vi "UHR-Fleezers Control (host) - 12.5.vi"() -> ()   [LabVIEW 2012] (continued)
                  n249 = And(x=w462, y=w459) -> (x .and. y?=w461:bool)
                  n250 = case "Only if were fishing and now formed tether" shown="False" w461 {
                    tunnel: w460 -> [w464 w479]
                    tunnel: [w463 w478] -> w458
                    tunnel: w457 -> [_ w474]
                    frame False {
                      n251 = local read "Fish for Tether"() -> (w463:bool)
                      n252 = case shown="False" w463 {
                        tunnel: w464 -> [w465 _]
                        frame False {
                          n253 = property on="BD 1 Frequency 1 (MHz)" class="DigNum (strict)"("Val(Sgnl)"=w465) -> ()  [unwired: 2 in, 2 out]
                        }
                        frame True {
                        }
                      }
                    }
                    frame True {
                      w478 = FALSE ("Fish for Tether")
                      n254 = call <vilib>:"Beep.vi"() -> ()  [unwired: 3 in, 9 out]
                      n255 = Number To Decimal String(number=w474, width (-)=i16 1) -> (decimal integer string=w472:string)
                      n256 = Concatenate Strings("Formed tether in ", w472, " attempt(s)." ("string")) -> (w469:string)
                      n257 = local read "Messages"() -> (w476:string)
                      n258 = local write "Fish for Tether"(w478) -> ()
                      n259 = call "Update messages.vi"("Message to add"=w469, "Old message string"=w476) -> ("New message string"=w475:string)
                      n260 = local write "Messages"(w475) -> ()
                      n261 = Get Date/Time In Seconds() -> (seconds since 1Jan1904=→"Time tether formed":timestamp)
                      n262 = local read "Flow ON during cal?"() -> (w466:bool)
                      n263 = property on="Sample Channel\nFlow" class="Bool (strict)"("Val(Sgnl)"=w466) -> (error out=w467:errorcluster)  [unwired: 2 in, 1 out]
                      n264 = case shown="\"2\", \"3\", \"4\", \"5\", \"6\"" "Then..." {
                        selector: "Then..." -> [_ w482]
                        tunnel: w479 -> [w481 _]
                        tunnel: w467 -> [_ _]
                        frame "1", Default {
                          n265 = property on="BD 1 Frequency 1 (MHz)" class="DigNum (strict)"("Val(Sgnl)"=w481) -> ()  [unwired: 2 in, 2 out]
                        }
                        frame "2", "3", "4", "5", "6" {
                          n266 = flat-sequence {
                            tunnel: w482 -> [w484]
                            frame #0 {
                              n267 = property on="Trap Delta (MHz)" class="DigNum (strict)"("Val(Sgnl)"="Move to Delta 1 (MHz)") -> ()  [unwired: 2 in, 2 out]
                            }
                            frame #1 {
                              n268 = case shown="\"5\", \"6\"" w484 {
                                selector: w484 -> [w487 w497 _]
                                frame "3", "4" {
                                n269 = flat-sequence {
                                tunnel: w487 -> [w488]
                                tunnel: [w488] -> w485
                                tunnel: [w490] -> w486
                                tunnel: w485 -> [w490]
                                tunnel: w486 -> [w494]
                                frame #0 {
                                n270 = property on="Green Laser ON" class="Bool (strict)"("Val(Sgnl)"=TRUE ("Value (Signaling)")) -> ()  [unwired: 2 in, 2 out]
                                }
                                frame #1 {
                                n271 = Multiply(x="Wait Before Save (s)", y=u32 1000 ("x")) -> (x*y=w492:u32)
                                n272 = Wait (ms)(milliseconds to wait=w492) -> ()  [unwired: 1 out]
                                }
                                frame #2 {
                                n273 = property on="Start Saving" class="Bool (strict)"("Value"=TRUE ("Start Saving")) -> ()  [unwired: 2 in, 2 out]
                                n274 = case shown="\"4\"" w494 {
                                frame Default {
                                }
                                frame "4" {
                                n275 = property on="Fl. Triggered..." class="Bool (strict)"("Val(Sgnl)"=TRUE ("Value (Signaling)")) -> ()  [unwired: 2 in, 2 out]
                                }
                                }
                                }
                                }
                                }
                                frame "5", "6" {
                                n276 = stacked-sequence {
                                tunnel: w497 -> [_ _ _ _ _ _ w509]
                                frame #0 {
                                n277 = Replace Array Subset(array=u32[] [0] ("Index Values"), new element="Raster Set Upon Tether", index=0) -> (w498:u32[])
                                n278 = property on="Saved AOD Raster Scan Parameter Sets" class="Arr (strict)"("Index Values"=w498) -> ()  [unwired: 2 in, 2 out]
                                }
                                frame #1 {
                                n279 = Wait (ms)(milliseconds to wait=u32 500) -> ()  [unwired: 1 out]
                                }
                                frame #2 {
                                n280 = property on="Load parameters" class="Bool (strict)"("Val(Sgnl)"=TRUE ("Value (Signaling)")) -> ()  [unwired: 2 in, 2 out]
                                n281 = case shown="True" "Green ON During Raster" {
                                frame False {
                                }
                                frame True {
                                n282 = property on="Green Laser ON" class="Bool (strict)"("Val(Sgnl)"=TRUE ("Value (Signaling)")) -> ()  [unwired: 2 in, 2 out]
                                }
                                }
                                }
                                frame #3 {
                                n283 = Wait (ms)(milliseconds to wait=u32 500) -> ()  [unwired: 1 out]
                                }
                                frame #4 {
                                n284 = property on="Trap Raster Scan" class="Bool (strict)"("Val(Sgnl)"=TRUE ("Value (Signaling)")) -> ()  [unwired: 2 in, 2 out]
                                }
                                frame #5 {
                                n285 = Wait (ms)(milliseconds to wait=u32 2000) -> ()  [unwired: 1 out]
                                }
                                frame #6 {
                                n286 = flat-sequence {
                                tunnel: w509 -> [w516]
                                frame #0 {
                                n287 = while {
                                stop <- w512 stop-if-true
                                n288 = local read "Raster Scanning..."() -> (w511:bool)
                                n289 = local read "Saving..."() -> (w514:bool)
                                n290 = Wait (ms)(milliseconds to wait=u32 100) -> ()  [unwired: 1 out]
                                n291 = Not(x=w514) -> (.not. x?=w513:bool)
                                n292 = Not(x=w511) -> (.not. x?=w510:bool)
                                n293 = And(x=w513, y=w510) -> (x .and. y?=w512:bool)
                                }
                                }
                                frame #1 {
                                n294 = local read "Tether"() -> (w517:bool)
                                n295 = case shown="True" w517 {
                                tunnel: w516 -> [_ w519]
                                frame False {
                                n296 = property on="Fish for Tether" class="Bool (strict)"("Val(Sgnl)"="Fish again after \nraster break?") -> ()  [unwired: 2 in, 2 out]
                                }
                                frame True {
                                n297 = stacked-sequence {
                                tunnel: w519 -> [_ w523 _ _]
                                frame #0 {
                                n298 = property on="Trap Delta (MHz)" class="DigNum (strict)"("Val(Sgnl)"="Move to Delta 2 (MHz)") -> ()  [unwired: 2 in, 2 out]
                                n299 = case shown="True" "Flow ON after\ntether testing?" {
                                frame False {
                                }
                                frame True {
                                n300 = property on="Sample Channel\nFlow" class="Bool (strict)"("Val(Sgnl)"=TRUE ("Value (Signaling)")) -> ()  [unwired: 2 in, 2 out]
                                }
                                }
                                }
                                frame #1 {
                                n301 = flat-sequence {
                                tunnel: w523 -> [w525]
                                frame #0 {
                                n302 = Wait (ms)(milliseconds to wait=u32 500) -> ()  [unwired: 1 out]
                                }
                                frame #1 {
                                n303 = case shown="\"6\"" w525 {
                                frame Default {
                                }
                                frame "6" {
                                n304 = property on="Green Laser ON" class="Bool (strict)"("Val(Sgnl)"=TRUE ("Green Laser ON/Interlacing")) -> ()  [unwired: 2 in, 2 out]
                                }
                                }
                                }
                                frame #2 {
                                n305 = Wait (ms)(milliseconds to wait=u32 500) -> ()  [unwired: 1 out]
                                }
                                frame #3 {
                                n306 = local write "Start Saving"("Save at end (5, 6)") -> ()
                                }
                                }
                                }
                                frame #2 {
                                n307 = local read "Bead Sep. Int. Time (s)"() -> (w531:dbl)
                                n308 = Multiply(x=w531, y=1000.0) -> (x*y=w530:dbl)
                                n309 = Wait (ms)(milliseconds to wait=w530) -> ()  [unwired: 1 out]
                                }
                                frame #3 {
                                n310 = property on="Remove Offset" class="Bool (strict)"("Val(Sgnl)"=TRUE ("Value (Signaling)")) -> ()  [unwired: 2 in, 2 out]
                                }
                                }
                                }
                                }
                                }
                                }
                                }
                                }
                                }
                                frame "2", Default {
                                }
                              }
                            }
                          }
                        }
                      }
                      "Tether" <- "Tether Alarm?"
                    }
                  }
                }
                frame #2 {
                  n311 = local read "Oscillate Set 1"() -> (w538:bool)
                  n312 = local read "Stop All"() -> (w536:bool)
                  n313 = Or(x=w538, y=w533) -> (x .or. y?=w535:bool)
                  n314 = Not(x=w535) -> (.not. x?=w537:bool)
                  n315 = Compound Arithmetic op=OR(w536, w537) -> (w534:bool)
                }
              }
              n316 = node-c288() -> ()  [unwired: 2 out]
            }
            n317 = node-c288(w379) -> ()  [unwired: 1 out]
          }
        }
      }
      event "Fl. Triggered...": Value Change {
        n318 = event-data() -> ()  [unwired: 7 out]
        n319 = case shown="True" "Fl. Triggered..." {
          frame False {
          }
          frame True {
            n320 = node-c288() -> (w549:T23)  [unwired: 4 out]
            n321 = timed-loop {
              timing: w549 -> [_]
              timing-out: [_] -> w548
              tunnel: "Action" -> [w557]
              shift-right: [w554] -> _
              shift-left: u8 255 -> [w556]
              shift-right: [w551] -> _
              shift-left: 255 -> [w553]
              stop <- w550 stop-if-true
              # "Reset confocal spot"
              n322 = node-c288() -> ()  [unwired: 2 out]
              n323 = flat-sequence {
                tunnel: w557 -> [w577]
                tunnel: w556 -> [w576]
                tunnel: [w575] -> w555
                tunnel: w553 -> [w562]
                tunnel: [w561] -> w552
                tunnel: [w956] -> w550
                tunnel: w555 -> [w955]
                tunnel: [w955] -> w554
                tunnel: [w954] -> w551
                tunnel: w552 -> [w954]
                frame #0 {
                  n324 = local read "Delta Fl. 2"() -> (w574:dbl)
                  n325 = local read "Delta Fl. 1"() -> (w569:dbl)
                  n326 = Multiply(x="Fl. Delta Thresh. (kHz)", y=1000.0) -> (x*y=w564:dbl)
                  n327 = Select(t=w569, s="APD to Watch", f=w574) -> (s? t:f=w565:dbl)
                  n328 = Greater?(x=w565, y=w564) -> (0:w570:bool)
                  n329 = Or(x="Force Yank", y=w570) -> (x .or. y?=w568:bool)
                  n330 = And(x=w568, y="Yank when?") -> (x .and. y?=w566:bool)
                  n331 = case shown="False" w566 {
                    tunnel: w577 -> [w580 w781]
                    tunnel: w576 -> [w582 w777]
                    tunnel: [w582 w775] -> w575
                    tunnel: w565 -> [w588 _]
                    tunnel: w564 -> [w587 _]
                    tunnel: "Force Yank" -> [w585 _]
                    tunnel: w562 -> [w584 w774]
                    tunnel: [w583 w774] -> w561
                    frame False {
                      n332 = Negate(x=w587) -> (-x=w579:dbl)
                      n333 = local write "Fl. High"(TRUE ("Fl. High")) -> ()
                      n334 = Less?(x=w588, y=w579) -> (x < y?=w586:bool)
                      n335 = Or(x=w585, y=w586) -> (x .or. y?=w581:bool)
                      n336 = case shown="True" w581 {
                        tunnel: w584 -> [w589 w599]
                        tunnel: [w589 w598] -> w583
                        tunnel: w580 -> [_ w597]
                        frame False {
                        }
                        frame True {
                          n337 = flat-sequence {
                            tunnel: w599 -> [w605]
                            tunnel: w597 -> [w602]
                            tunnel: [w604] -> w596
                            tunnel: [w603] -> w595
                            tunnel: [w602] -> w594
                            tunnel: w593 -> [w601]
                            tunnel: [w601] -> w592
                            tunnel: w591 -> [w600]
                            tunnel: [w600] -> w590
                            tunnel: [w676] -> w598
                            tunnel: w596 -> [w676]
                            tunnel: w595 -> [w675]
                            tunnel: w594 -> [w674]
                            tunnel: w592 -> [w673]
                            tunnel: w590 -> [w672]
                            frame #0 {
                              n338 = call <vilib>:"Beep.vi"() -> ()  [unwired: 12 in]
                              n339 = local write "Waiting"(FALSE ("Waiting")) -> ()
                              n340 = Increment(x=w605) -> (x+1=w604:i32)
                              n341 = case shown="\"Image\"" w602 {
                                tunnel: w604 -> [_ w610 _]
                                frame "Alarm", Default {
                                }
                                frame "Yank" {
                                n342 = flat-sequence {
                                tunnel: w610 -> [w613]
                                tunnel: [w612] -> w609
                                tunnel: [w611] -> w608
                                tunnel: w609 -> [w623]
                                tunnel: w608 -> [w624]
                                frame #0 {
                                n343 = local read "Yank Delay (s)"() -> (w616:dbl)
                                n344 = local read "N Array El"() -> (w611:u8)
                                n345 = Quotient & Remainder(x=w613, y=w611) -> (x-y*floor(x/y)=w612:i32)  [unwired: 1 out]
                                n346 = Multiply(x=w616, y=1000.0) -> (x*y=w614:dbl)
                                n347 = Wait (ms)(milliseconds to wait=w614) -> ()  [unwired: 1 out]
                                }
                                frame #1 {
                                n348 = local read "Yank to which?"() -> (w618:bool)
                                n349 = local read "Random Choice"() -> (w628:bool)
                                n350 = local read "Yank to Trap Delta (MHz)"() -> (w621:dbl[])
                                n351 = local read "Yank to SP"() -> (w622:dbl[])
                                n352 = Random Number (0-1)() -> (number: 0 to 1=w627:dbl)
                                n353 = Multiply(x=w624, y=w627) -> (x*y=w626:dbl)
                                n354 = Round Toward -Infinity(1:w626) -> (0:w625:dbl)
                                n355 = Select(t=w625, s=w628, f=w623) -> (s? t:f=w619:dbl)
                                n356 = Select(t=w621, s=w618, f=w622) -> (s? t:f=w620:dbl[])
                                n357 = Index Array(array=w620, index=w619) -> (element=w617:dbl)
                                n358 = case shown="True" w618 {
                                tunnel: w617 -> [w629 w656]
                                frame False {
                                n359 = flat-sequence {
                                tunnel: w629 -> [w630]
                                frame #0 {
                                n360 = property on="Trap Pos FB SP" class="DigNum (strict)"("Val(Sgnl)"=w630) -> ()  [unwired: 2 in, 2 out]
                                }
                                frame #1 {
                                n361 = Wait (ms)(milliseconds to wait=u32 700) -> ()  [unwired: 1 out]
                                }
                                frame #2 {
                                n362 = local read "Action (%)"() -> (w635:dbl)
                                n363 = Absolute Value(x=w635) -> (abs(x)=w634:dbl)
                                n364 = Greater?(x=w634, y=70.0) -> (0:w632:bool)
                                n365 = property on="Remove Action Offset" class="Bool (strict)"("Val(Sgnl)"=w632) -> ()  [unwired: 2 in, 2 out]
                                }
                                frame #3 {
                                n366 = for {
                                N: 4 -> [_]
                                n367 = flat-sequence {
                                frame #0 {
                                n368 = Wait (ms)(milliseconds to wait=u32 500) -> ()  [unwired: 1 out]
                                }
                                frame #1 {
                                n369 = local read "Action (%)"() -> (w641:dbl)
                                n370 = Absolute Value(x=w641) -> (abs(x)=w640:dbl)
                                n371 = Greater?(x=w640, y=70.0) -> (0:w638:bool)
                                n372 = property on="Remove Action Offset" class="Bool (strict)"("Val(Sgnl)"=w638) -> ()  [unwired: 2 in, 2 out]
                                }
                                }
                                }
                                }
                                frame #4 {
                                n373 = Wait (ms)(milliseconds to wait=u32 500) -> ()  [unwired: 1 out]
                                }
                                frame #5 {
                                n374 = local read "Mean"() -> (w649:dbl)
                                n375 = Greater?(x=w649, y=11.0) -> (0:w643:bool)
                                n376 = Not(x=w643) -> (.not. x?=w644:bool)
                                n377 = And(x=w644, y="Shift confocal") -> (x .and. y?=w646:bool)
                                n378 = And(x=w643, y="Shift confocal") -> (x .and. y?=w647:bool)
                                n379 = case shown="True" w647 {
                                frame False {
                                }
                                frame True {
                                n380 = local read "Confocal Y 2 (V)"() -> (w653:dbl)
                                n381 = local read "Confocal X 2 (V)"() -> (w652:dbl)
                                n382 = property on="AO1" class="Slide (strict)"("Val(Sgnl)"=w653) -> ()  [unwired: 2 in, 2 out]
                                n383 = property on="AO2" class="Slide (strict)"("Val(Sgnl)"=w652) -> ()  [unwired: 2 in, 2 out]
                                }
                                }
                                n384 = case shown="True" w646 {
                                frame False {
                                }
                                frame True {
                                n385 = local read "Confocal Y 1 (V)"() -> (w651:dbl)
                                n386 = local read "Confocal X 1 (V)"() -> (w650:dbl)
                                n387 = property on="AO1" class="Slide (strict)"("Val(Sgnl)"=w651) -> ()  [unwired: 2 in, 2 out]
                                n388 = property on="AO2" class="Slide (strict)"("Val(Sgnl)"=w650) -> ()  [unwired: 2 in, 2 out]
                                }
                                }
                                }
                                frame #6 {
                                n389 = Wait (ms)(milliseconds to wait=u32 1500) -> ()  [unwired: 1 out]
                                }
                                frame #7 {
                                n390 = property on="Rem fb disp offset" class="Bool (strict)"("Val(Sgnl)"=TRUE ("Value (Signaling)")) -> ()  [unwired: 2 in, 2 out]
                                }
                                }
                                }
                                frame True {
                                n391 = flat-sequence {
                                tunnel: w656 -> [w657]
                                frame #0 {
                                n392 = property on="Trap Delta (MHz)" class="DigNum (strict)"("Val(Sgnl)"=w657) -> ()  [unwired: 2 in, 2 out]
                                }
                                frame #1 {
                                n393 = Wait (ms)(milliseconds to wait=u32 500) -> ()  [unwired: 1 out]
                                }
                                frame #2 {
                                n394 = local read "Shift confocal"() -> (w663:bool)
                                n395 = local read "Mean"() -> (w665:dbl)
                                n396 = Greater?(x=w665, y=11.0) -> (0:w662:bool)
                                n397 = Not(x=w662) -> (.not. x?=w661:bool)
                                n398 = And(x=w661, y=w663) -> (x .and. y?=w659:bool)
                                n399 = And(x=w662, y=w663) -> (x .and. y?=w660:bool)
                                n400 = case shown="True" w660 {
                                frame False {
                                }
                                frame True {
                                n401 = local read "Confocal Y 2 (V)"() -> (w669:dbl)
                                n402 = local read "Confocal X 2 (V)"() -> (w668:dbl)
                                n403 = property on="AO2" class="Slide (strict)"("Val(Sgnl)"=w668) -> ()  [unwired: 2 in, 2 out]
                                n404 = property on="AO1" class="Slide (strict)"("Val(Sgnl)"=w669) -> ()  [unwired: 2 in, 2 out]
                                }
                                }
                                n405 = case shown="True" w659 {
                                frame False {
                                }
                                frame True {
                                n406 = local read "Confocal X 1 (V)"() -> (w666:dbl)
                                n407 = local read "Confocal Y 1 (V)"() -> (w667:dbl)
                                n408 = property on="AO2" class="Slide (strict)"("Val(Sgnl)"=w666) -> ()  [unwired: 2 in, 2 out]
                                n409 = property on="AO1" class="Slide (strict)"("Val(Sgnl)"=w667) -> ()  [unwired: 2 in, 2 out]
                                }
                                }
                                }
                                }
                                }
                                }
                                }
                                }
                                }
                                frame "Image" {
                                n410 = property on="Confocal Image" class="Bool (strict)"("Val(Sgnl)"=TRUE ("Value (Signaling)")) -> ()  [unwired: 2 in, 2 out]
                                }
                              }
                              n411 = local write "Fl. High"(FALSE ("Fl. High")) -> ()
                              n412 = local read "Time (s)"() -> (w603:dbl)
                            }
                            frame #1 {
                              n413 = case shown="True" "Auto F Reset" {
                                tunnel: w675 -> [_ w680]
                                tunnel: w674 -> [_ w679]
                                tunnel: w673 -> [_ w678]
                                tunnel: w672 -> [_ w677]
                                frame False {
                                }
                                frame True {
                                n414 = node-c288() -> (w682:T23)  [unwired: 4 in]
                                n415 = timed-loop {
                                timing: w682 -> [_]
                                timing-out: [_] -> w681
                                tunnel: w680 -> [w687]
                                tunnel: w679 -> [w686]
                                tunnel: w678 -> [w685]
                                tunnel: w677 -> [w684]
                                stop <- w683 stop-if-true
                                n416 = node-c288() -> ()  [unwired: 1 in, 1 out]
                                n417 = local read "Fl. Delta Thresh. (kHz)"() -> (w696:dbl)
                                n418 = local read "APD to Watch"() -> (w697:bool)
                                n419 = local read "Delta Fl. 1"() -> (w698:dbl)
                                n420 = local read "Delta Fl. 2"() -> (w699:dbl)
                                n421 = local read "Fl. Triggered..."() -> (w690:bool)
                                n422 = local read "Stop All"() -> (w691:bool)
                                n423 = local read "Reset Force"() -> (w689:bool)
                                n424 = Multiply(x=w696, y=1000.0) -> (x*y=w694:dbl)
                                n425 = Select(t=w698, s=w697, f=w699) -> (s? t:f=w693:dbl)
                                n426 = Not(x=w690) -> (.not. x?=w688:bool)
                                n427 = Greater?(x=w693, y=w694) -> (0:w692:bool)
                                n428 = Compound Arithmetic op=OR(w692, w691, w688, w689) -> (w683:bool)
                                n429 = case shown="True" w683 {
                                tunnel: w687 -> [_ w703]
                                tunnel: w686 -> [_ w707]
                                tunnel: w685 -> [_ w706]
                                tunnel: w684 -> [_ w705]
                                frame False {
                                }
                                frame True {
                                n430 = case shown="\"Yank\"" w707 {
                                tunnel: w706 -> [_ w717]
                                tunnel: w705 -> [_ w715]
                                frame "Image", Default {
                                }
                                frame "Yank" {
                                n431 = flat-sequence {
                                tunnel: [w720] -> w718
                                tunnel: w717 -> [w720]
                                tunnel: [w719] -> w716
                                tunnel: w715 -> [w719]
                                tunnel: w718 -> [w726]
                                tunnel: w716 -> [w724]
                                frame #0 {
                                n432 = local read "Yank Delay (s)"() -> (w723:dbl)
                                n433 = Multiply(x=w723, y=1000.0) -> (x*y=w721:dbl)
                                n434 = Wait (ms)(milliseconds to wait=w721) -> ()  [unwired: 1 out]
                                }
                                frame #1 {
                                n435 = local read "Yank to which?"() -> (w725:bool)
                                n436 = case shown="False" w725 {
                                tunnel: w726 -> [_ w754]
                                tunnel: w724 -> [w727 _]
                                frame False {
                                n437 = flat-sequence {
                                tunnel: w727 -> [w728]
                                frame #0 {
                                n438 = property on="Trap Pos FB SP" class="DigNum (strict)"("Val(Sgnl)"=w728) -> ()  [unwired: 2 in, 2 out]
                                }
                                frame #1 {
                                n439 = Wait (ms)(milliseconds to wait=u32 700) -> ()  [unwired: 1 out]
                                }
                                frame #2 {
                                n440 = local read "Action (%)"() -> (w733:dbl)
                                n441 = Absolute Value(x=w733) -> (abs(x)=w732:dbl)
                                n442 = Greater?(x=w732, y=70.0) -> (0:w730:bool)
                                n443 = property on="Remove Action Offset" class="Bool (strict)"("Val(Sgnl)"=w730) -> ()  [unwired: 2 in, 2 out]
                                }
                                frame #3 {
                                n444 = for {
                                N: 4 -> [_]
                                n445 = flat-sequence {
                                frame #0 {
                                n446 = Wait (ms)(milliseconds to wait=u32 500) -> ()  [unwired: 1 out]
                                }
                                frame #1 {
                                n447 = local read "Action (%)"() -> (w739:dbl)
                                n448 = Absolute Value(x=w739) -> (abs(x)=w738:dbl)
                                n449 = Greater?(x=w738, y=70.0) -> (0:w736:bool)
                                n450 = property on="Remove Action Offset" class="Bool (strict)"("Val(Sgnl)"=w736) -> ()  [unwired: 2 in, 2 out]
                                }
                                }
                                }
                                }
                                frame #4 {
                                n451 = Wait (ms)(milliseconds to wait=u32 500) -> ()  [unwired: 1 out]
                                }
                                frame #5 {
                                n452 = local read "Shift confocal"() -> (w744:bool)
                                n453 = local read "Mean"() -> (w747:dbl)
                                n454 = Greater?(x=w747, y=11.0) -> (0:w743:bool)
                                n455 = Not(x=w743) -> (.not. x?=w742:bool)
                                n456 = And(x=w743, y=w744) -> (x .and. y?=w745:bool)
                                n457 = And(x=w742, y=w744) -> (x .and. y?=w741:bool)
                                n458 = case shown="True" w745 {
                                frame False {
                                }
                                frame True {
                                n459 = local read "Confocal X 2 (V)"() -> (w750:dbl)
                                n460 = local read "Confocal Y 2 (V)"() -> (w751:dbl)
                                n461 = property on="AO2" class="Slide (strict)"("Val(Sgnl)"=w750) -> ()  [unwired: 2 in, 2 out]
                                n462 = property on="AO1" class="Slide (strict)"("Val(Sgnl)"=w751) -> ()  [unwired: 2 in, 2 out]
                                }
                                }
                                n463 = case shown="True" w741 {
                                frame False {
                                }
                                frame True {
                                n464 = local read "Confocal Y 1 (V)"() -> (w749:dbl)
                                n465 = local read "Confocal X 1 (V)"() -> (w748:dbl)
                                n466 = property on="AO1" class="Slide (strict)"("Val(Sgnl)"=w749) -> ()  [unwired: 2 in, 2 out]
                                n467 = property on="AO2" class="Slide (strict)"("Val(Sgnl)"=w748) -> ()  [unwired: 2 in, 2 out]
                                }
                                }
                                }
                                frame #6 {
                                n468 = Wait (ms)(milliseconds to wait=u32 1500) -> ()  [unwired: 1 out]
                                }
                                frame #7 {
                                n469 = property on="Rem fb disp offset" class="Bool (strict)"("Val(Sgnl)"=TRUE ("Value (Signaling)")) -> ()  [unwired: 2 in, 2 out]
                                }
                                }
                                }
                                frame True {
                                n470 = flat-sequence {
                                tunnel: w754 -> [w755]
                                frame #0 {
                                n471 = property on="Trap Delta (MHz)" class="DigNum (strict)"("Val(Sgnl)"=w755) -> ()  [unwired: 2 in, 2 out]
                                }
                                frame #1 {
                                n472 = Wait (ms)(milliseconds to wait=u32 500) -> ()  [unwired: 1 out]
                                }
                                frame #2 {
                                n473 = local read "Shift confocal"() -> (w761:bool)
                                n474 = local read "Mean"() -> (w762:dbl)
                                n475 = Greater?(x=w762, y=11.0) -> (0:w760:bool)
                                n476 = And(x=w760, y=w761) -> (x .and. y?=w758:bool)
                                n477 = Not(x=w760) -> (.not. x?=w759:bool)
                                n478 = And(x=w759, y=w761) -> (x .and. y?=w757:bool)
                                n479 = case shown="True" w758 {
                                frame False {
                                }
                                frame True {
                                n480 = local read "Confocal Y 2 (V)"() -> (w767:dbl)
                                n481 = local read "Confocal X 2 (V)"() -> (w766:dbl)
                                n482 = property on="AO1" class="Slide (strict)"("Val(Sgnl)"=w767) -> ()  [unwired: 2 in, 2 out]
                                n483 = property on="AO2" class="Slide (strict)"("Val(Sgnl)"=w766) -> ()  [unwired: 2 in, 2 out]
                                }
                                }
                                n484 = case shown="True" w757 {
                                frame False {
                                }
                                frame True {
                                n485 = local read "Confocal Y 1 (V)"() -> (w765:dbl)
                                n486 = local read "Confocal X 1 (V)"() -> (w764:dbl)
                                n487 = property on="AO2" class="Slide (strict)"("Val(Sgnl)"=w764) -> ()  [unwired: 2 in, 2 out]
                                n488 = property on="AO1" class="Slide (strict)"("Val(Sgnl)"=w765) -> ()  [unwired: 2 in, 2 out]
                                }
                                }
                                }
                                }
                                }
                                }
                                }
                                }
                                }
                                }
                                n489 = local read "Time (s)"() -> (w702:dbl)
                                n490 = Subtract(x=w703, y=w702) -> (x-y=w714:dbl)
                                n491 = Number To Decimal String(number=w714, width (-)=i16 0) -> (decimal integer string=w712:string)
                                n492 = Concatenate Strings(w712, " s fluorescence event") -> (w709:string)
                                n493 = local read "Messages"() -> (w710:string)
                                n494 = local write "Duration (s)"(w714) -> ()
                                n495 = call "Update messages.vi"("Message to add"=w709, "Old message string"=w710) -> ("New message string"=w708:string)
                                n496 = local write "Messages"(w708) -> ()
                                n497 = call <vilib>:"Beep.vi"() -> ()  [unwired: 12 in]
                                n498 = local write "Reset Force"(FALSE ("Force Reset")) -> ()
                                n499 = local write "Fl. High"(TRUE ("Fl. High")) -> ()
                                n500 = local write "Waiting"(TRUE ("Waiting")) -> ()
                                }
                                }
                                n501 = node-c288() -> ()  [unwired: 1 in, 1 out]
                                }
                                n502 = node-c288(w681) -> ()  [unwired: 1 out]
                                }
                              }
                            }
                          }
                          n503 = local read "Trap Delta (MHz)"() -> (w593:dbl)
                          n504 = local read "Trap Pos FB SP"() -> (w591:fxp<+/-,16,1>)
                        }
                      }
                    }
                    frame True {
                      n505 = flat-sequence {
                        tunnel: w778 -> [w788]
                        tunnel: [w788] -> w782
                        tunnel: w781 -> [w787]
                        tunnel: [w787] -> w780
                        tunnel: [w786] -> w779
                        tunnel: w777 -> [w785]
                        tunnel: [w784] -> w776
                        tunnel: w773 -> [w783]
                        tunnel: [w783] -> w772
                        tunnel: w782 -> [w858]
                        tunnel: w780 -> [w857]
                        tunnel: w779 -> [w856]
                        tunnel: w776 -> [w855]
                        tunnel: w772 -> [w854]
                        tunnel: [w855] -> w775
                        frame #0 {
                          n506 = call <vilib>:"Beep.vi"() -> ()  [unwired: 3 in, 9 out]
                          n507 = local write "Waiting"(FALSE ("Waiting")) -> ()
                          n508 = Increment(x=w785) -> (x+1=w784:u8)
                          n509 = case shown="\"Yank\"" w787 {
                            tunnel: w784 -> [_ _ w794]
                            frame "Image" {
                              n510 = property on="Confocal Image" class="Bool (strict)"("Val(Sgnl)"=TRUE ("Value (Signaling)")) -> ()  [unwired: 2 in, 2 out]
                            }
                            frame "Alarm", Default {
                            }
                            frame "Yank" {
                              n511 = flat-sequence {
                                tunnel: w794 -> [w797]
                                tunnel: [w796] -> w793
                                tunnel: ["N Array El"] -> w792
                                tunnel: w793 -> [w811]
                                tunnel: w792 -> [w807]
                                frame #0 {
                                n512 = Multiply(x="Yank Delay (s)", y=1000.0) -> (x*y=w800:dbl)
                                n513 = Quotient & Remainder(x=w797, y="N Array El") -> (x-y*floor(x/y)=w796:u8)  [unwired: 1 out]
                                n514 = Wait (ms)(milliseconds to wait=w800) -> ()  [unwired: 1 out]
                                }
                                frame #1 {
                                n515 = Random Number (0-1)() -> (number: 0 to 1=w808:dbl)
                                n516 = Multiply(x=w807, y=w808) -> (x*y=w806:dbl)
                                n517 = Round Toward -Infinity(1:w806) -> (0:w805:dbl)
                                n518 = Select(t=w805, s="Random Choice", f=w811) -> (s? t:f=w809:dbl)
                                n519 = Select(t="Yank to Trap Delta (MHz)", s="Yank to which?", f="Yank to SP") -> (s? t:f=w802:dbl[])
                                n520 = Index Array(array=w802, index=w809) -> (element=w812:dbl)
                                n521 = case shown="False" "Yank to which?" {
                                tunnel: w812 -> [w813 w839]
                                frame False {
                                n522 = flat-sequence {
                                tunnel: w813 -> [w814]
                                frame #0 {
                                n523 = property on="Trap Pos FB SP" class="DigNum (strict)"("Val(Sgnl)"=w814) -> ()  [unwired: 2 in, 2 out]
                                }
                                frame #1 {
                                n524 = Wait (ms)(milliseconds to wait=u32 700) -> ()  [unwired: 1 out]
                                }
                                frame #2 {
                                n525 = local read "Action (%)"() -> (w819:dbl)
                                n526 = Absolute Value(x=w819) -> (abs(x)=w818:dbl)
                                n527 = Greater?(x=w818, y=70.0) -> (0:w816:bool)
                                n528 = property on="Remove Action Offset" class="Bool (strict)"("Val(Sgnl)"=w816) -> ()  [unwired: 2 in, 2 out]
                                }
                                frame #3 {
                                n529 = for {
                                N: 4 -> [_]
                                n530 = flat-sequence {
                                frame #0 {
                                n531 = Wait (ms)(milliseconds to wait=u32 500) -> ()  [unwired: 1 out]
                                }
                                frame #1 {
                                n532 = local read "Action (%)"() -> (w825:dbl)
                                n533 = Absolute Value(x=w825) -> (abs(x)=w824:dbl)
                                n534 = Greater?(x=w824, y=70.0) -> (0:w822:bool)
                                n535 = property on="Remove Action Offset" class="Bool (strict)"("Val(Sgnl)"=w822) -> ()  [unwired: 2 in, 2 out]
                                }
                                }
                                }
                                }
                                frame #4 {
                                n536 = local read "Shift confocal"() -> (w829:bool)
                                n537 = local read "Mean"() -> (w832:dbl)
                                n538 = Greater?(x=w832, y=11.0) -> (0:w828:bool)
                                n539 = Not(x=w828) -> (.not. x?=w827:bool)
                                n540 = And(x=w827, y=w829) -> (x .and. y?=w826:bool)
                                n541 = And(x=w828, y=w829) -> (x .and. y?=w830:bool)
                                n542 = case shown="True" w830 {
                                frame False {
                                }
                                frame True {
                                n543 = local read "Confocal X 2 (V)"() -> (w835:dbl)
                                n544 = local read "Confocal Y 2 (V)"() -> (w836:dbl)
                                n545 = property on="AO2" class="Slide (strict)"("Val(Sgnl)"=w835) -> ()  [unwired: 2 in, 2 out]
                                n546 = property on="AO1" class="Slide (strict)"("Val(Sgnl)"=w836) -> ()  [unwired: 2 in, 2 out]
                                }
                                }
                                n547 = case shown="True" w826 {
                                frame False {
                                }
                                frame True {
                                n548 = local read "Confocal X 1 (V)"() -> (w833:dbl)
                                n549 = local read "Confocal Y 1 (V)"() -> (w834:dbl)
                                n550 = property on="AO1" class="Slide (strict)"("Val(Sgnl)"=w834) -> ()  [unwired: 2 in, 2 out]
                                n551 = property on="AO2" class="Slide (strict)"("Val(Sgnl)"=w833) -> ()  [unwired: 2 in, 2 out]
                                }
                                }
                                }
                                frame #5 {
                                n552 = Wait (ms)(milliseconds to wait=u32 1500) -> ()  [unwired: 1 out]
                                }
                                frame #6 {
                                n553 = property on="Rem fb disp offset" class="Bool (strict)"("Val(Sgnl)"=TRUE ("Value (Signaling)")) -> ()  [unwired: 2 in, 2 out]
                                }
                                }
                                }
                                frame True {
                                n554 = flat-sequence {
                                tunnel: w839 -> [w840]
                                frame #0 {
                                n555 = property on="Trap Delta (MHz)" class="DigNum (strict)"("Val(Sgnl)"=w840) -> ()  [unwired: 2 in, 2 out]
                                }
                                frame #1 {
                                n556 = Wait (ms)(milliseconds to wait=u32 500) -> ()  [unwired: 1 out]
                                }
                                frame #2 {
                                n557 = local read "Shift confocal"() -> (w844:bool)
                                n558 = local read "Mean"() -> (w842:dbl)
                                n559 = Greater?(x=w842, y=11.0) -> (0:w845:bool)
                                n560 = Not(x=w845) -> (.not. x?=w846:bool)
                                n561 = And(x=w846, y=w844) -> (x .and. y?=w848:bool)
                                n562 = And(x=w845, y=w844) -> (x .and. y?=w847:bool)
                                n563 = case shown="True" w847 {
                                frame False {
                                }
                                frame True {
                                n564 = local read "Confocal Y 2 (V)"() -> (w852:dbl)
                                n565 = local read "Confocal X 2 (V)"() -> (w851:dbl)
                                n566 = property on="AO1" class="Slide (strict)"("Val(Sgnl)"=w852) -> ()  [unwired: 2 in, 2 out]
                                n567 = property on="AO2" class="Slide (strict)"("Val(Sgnl)"=w851) -> ()  [unwired: 2 in, 2 out]
                                }
                                }
                                n568 = case shown="True" w848 {
                                frame False {
                                }
                                frame True {
                                n569 = local read "Confocal X 1 (V)"() -> (w849:dbl)
                                n570 = local read "Confocal Y 1 (V)"() -> (w850:dbl)
                                n571 = property on="AO2" class="Slide (strict)"("Val(Sgnl)"=w849) -> ()  [unwired: 2 in, 2 out]
                                n572 = property on="AO1" class="Slide (strict)"("Val(Sgnl)"=w850) -> ()  [unwired: 2 in, 2 out]
                                }
                                }
                                }
                                }
                                }
                                }
                                }
                              }
                            }
                          }
                          n573 = local read "Time (s)"() -> (w786:dbl)
                          "Fl. High" <- TRUE ("Yanking")
                        }
                        frame #1 {
                          n574 = local read "Auto F Reset"() -> (w853:bool)
                          n575 = case shown="True" w853 {
                            tunnel: w858 -> [_ w862]
                            tunnel: w857 -> [_ w861]
                            tunnel: w856 -> [_ w860]
                            tunnel: w854 -> [_ w859]
                            frame False {
                            }
                            frame True {
                              n576 = node-c288() -> (w864:T23)  [unwired: 4 out]
                              n577 = timed-loop {
                                timing: w864 -> [_]
                                timing-out: [_] -> w863
                                tunnel: w862 -> [w882]
                                tunnel: w861 -> [w881]
                                tunnel: w860 -> [w880]
                                tunnel: w859 -> [w879]
                                stop <- w865 stop-if-true
                                n578 = node-c288() -> ()  [unwired: 2 out]
                                n579 = local read "Fl. Delta Thresh. (kHz)"() -> (w873:dbl)
                                n580 = local read "Fl. Triggered..."() -> (w878:bool)
                                n581 = local read "Delta Fl. 1"() -> (w869:dbl)
                                n582 = local read "Delta Fl. 2"() -> (w867:dbl)
                                n583 = local read "Stop All"() -> (w876:bool)
                                n584 = local read "APD to Watch"() -> (w868:bool)
                                n585 = Select(t=w869, s=w868, f=w867) -> (s? t:f=w866:dbl)
                                n586 = Not(x=w878) -> (.not. x?=w877:bool)
                                n587 = Multiply(x=w873, y=1000.0) -> (x*y=w872:dbl)
                                n588 = Negate(x=w872) -> (-x=w871:dbl)
                                n589 = Less?(x=w866, y=w871) -> (x < y?=w875:bool)
                                n590 = Compound Arithmetic op=OR(w875, w876, w877, "Reset Force") -> (w865:bool)
                                n591 = case shown="True" w865 {
                                tunnel: w882 -> [_ w897]
                                tunnel: w881 -> [_ w896]
                                tunnel: w880 -> [_ w886]
                                tunnel: w879 -> [_ w888]
                                frame False {
                                }
                                frame True {
                                n592 = local read "Time (s)"() -> (w887:dbl)
                                n593 = case shown="\"Yank\"" w896 {
                                tunnel: w897 -> [_ w900]
                                tunnel: w888 -> [_ w898]
                                frame "Image", Default {
                                }
                                frame "Yank" {
                                n594 = flat-sequence {
                                tunnel: [w906] -> w901
                                tunnel: w900 -> [w906]
                                tunnel: [w902] -> w899
                                tunnel: w898 -> [w902]
                                tunnel: w901 -> [w909]
                                tunnel: w899 -> [w907]
                                frame #0 {
                                n595 = local read "Yank Delay (s)"() -> (w905:dbl)
                                n596 = Multiply(x=w905, y=1000.0) -> (x*y=w903:dbl)
                                n597 = Wait (ms)(milliseconds to wait=w903) -> ()  [unwired: 1 out]
                                }
                                frame #1 {
                                n598 = local read "Yank to which?"() -> (w908:bool)
                                n599 = case shown="False" w908 {
                                tunnel: w909 -> [_ w936]
                                tunnel: w907 -> [w910 _]
                                frame False {
                                n600 = flat-sequence {
                                tunnel: w910 -> [w911]
                                frame #0 {
                                n601 = property on="Trap Pos FB SP" class="DigNum (strict)"("Val(Sgnl)"=w911) -> ()  [unwired: 2 in, 2 out]
                                }
                                frame #1 {
